vi "testNoError.vi"() -> (0 "error out":errorcluster)   [LabVIEW 2017, in "Fact.Tests.lvlib"]
uses:
  Fact.Tests.lvlib
  Fact/Fact.lvclass
  Support/Support.lvlib
  Assertion/Assertion.lvlib
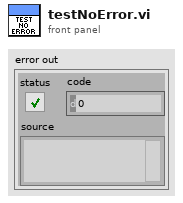
[diagram p1: front panel]
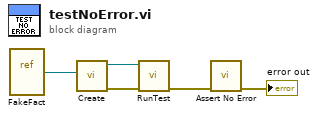
[diagram p0: block diagram]
diagram:
  n1 = vi-ref "FakeFact.vi"() -> (w1:refnum<vi>)
  n2 = call "Create.vi"("VI Refnum"=w1) -> ("error out"=w4:errorcluster, "Fact"=w5:refnum<class "Fact.lvclass">)  [unwired: 9 in]
  n3 = call-dynamic "RunTest.vi"("error in (no error)"=w4, "Fact in"=w5) -> ("error out"=w3:errorcluster)  [unwired: 8 in, 1 out]
  n4 = call "Assert No Error.vi"("error in (no error)"=w3) -> ("error out"=→"error out":errorcluster)  [unwired: 10 in]
